vi "Check Supports.vi"(8 "error in (no error)":errorcluster, 10 "Ctl Refnum":refnum<vi>, 11 "Element Filter in":refnum<class "Element Filter.lvclass">) -> (0 "error out":errorcluster, 2 "Supported":bool)   [LabVIEW 2020, in "Aether Engine.lvlib" / "Element Filter.lvclass"]
uses:
  Element Filter.lvclass
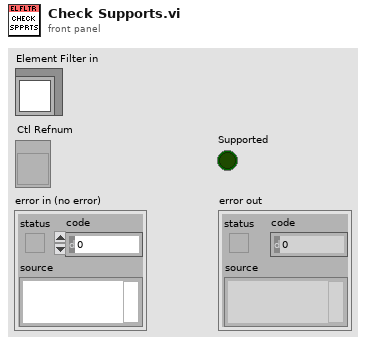
[diagram p1: front panel]
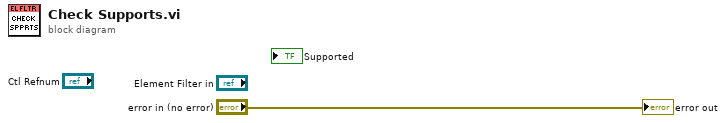
[diagram p0: block diagram]
diagram:
  "error out" <- "error in (no error)"
